vi "DT Read Encode.vi"(11 "Reset Encoders":bool) -> (2 "Drivetrain Encoder Values":T1)   [LabVIEW 2017]
uses:
  Common Code/Drivetrain Encoder Values.ctl
  Common Code/DT Encoder Values.ctl
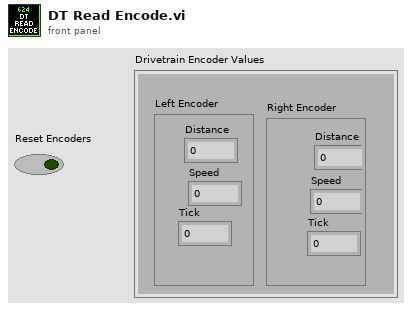
[diagram p1: front panel]
types:
  T1 = typedef "Drivetrain Encoder Values.ctl" = cluster{"Left Encoder":cluster{"Distance":dbl, "Speed":dbl, "Tick":dbl}, "Right Encoder":cluster{"Distance":dbl, "Speed":dbl, "Tick":dbl}}
  T2 = typedef "DT Encoder Values.ctl" = cluster{"Left Encoder":cluster{"Distance":dbl, "Speed":dbl, "Tick":dbl}, "Right Encoder":cluster{"Distance":dbl, "Speed":dbl, "Tick":dbl}}
  T3 = typedef "WPI_EncoderDevRef.ctl" = cluster{"DevStatus":errorcluster, "EncoderIndex":T4, "CounterIndex":T5, "DistancePerCount":dbl, "Decoding Type":T6}
  T4 = typedef "FPGA_EncoderIdx.ctl" = enum8{"Enc 0", "Enc 1", "Enc 2", "Enc 3", "Enc 4", "Enc 5", "Enc 6", "Enc 7", "Invalid"}
  T5 = typedef "FPGA_CounterCtrSystemIndex.ctl" = enum8{"Ctr 0", "Ctr 1", "Ctr 2", "Ctr 3", "Ctr 4", "Ctr 5", "Ctr 6", "Ctr 7", "Invalid"}
  T6 = typedef "WPI_EncoderType.ctl" = enum16{"1x", "2x", "4x"}
  T7 = typedef "Encoder Values.ctl" = cluster{"Distance":dbl, "Speed":dbl, "Tick":dbl}
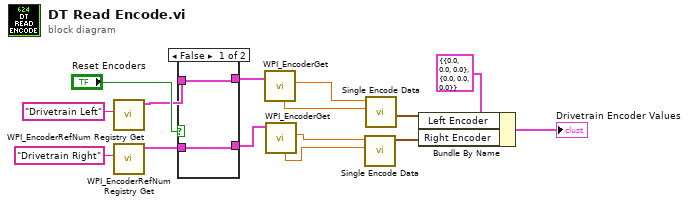
[diagram p0: block diagram]
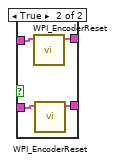
[diagram p2: hidden frame]
diagram:
  n1 = call <vilib>:"WPI_EncoderRefNum Registry Get.vi"("refnum name"="Drivetrain Left") -> ("EncoderDevRef"=w12:T3)  [unwired: 9 in, 1 out]
  n2 = call <vilib>:"WPI_EncoderRefNum Registry Get.vi"("refnum name"="Drivetrain Right") -> ("EncoderDevRef"=w11:T3)  [unwired: 9 in, 1 out]
  n3 = case shown="False" "Reset Encoders" {
    tunnel: w12 -> [w17 w21]
    tunnel: w11 -> [w16 w20]
    tunnel: [w17 w19] -> w10
    tunnel: [w16 w18] -> w9
    frame False {
    }
    frame True {
      n4 = call <vilib>:"WPI_EncoderReset.vi"("EncoderDevRef"=w21) -> ("EncoderDevRef"=w19:T3)  [unwired: 9 in, 1 out]
      n5 = call <vilib>:"WPI_EncoderReset.vi"("EncoderDevRef"=w20) -> ("EncoderDevRef"=w18:T3)  [unwired: 9 in, 1 out]
    }
  }
  n6 = call <vilib>:"WPI_EncoderGet.vi"("EncoderDevRef"=w10) -> ("Distance"=w5:dbl, "Rate"=w6:dbl)  [unwired: 5 in, 4 out]
  n7 = call <vilib>:"WPI_EncoderGet.vi"("EncoderDevRef"=w9) -> ("Distance"=w7:dbl, "Rate"=w8:dbl)  [unwired: 5 in, 4 out]
  n8 = call "Single Encode Data.vi"("Rate"=w8, "Distance"=w7) -> ("Encoder Values"=w2:T7)  [unwired: 9 in]
  n9 = call "Single Encode Data.vi"("Rate"=w6, "Distance"=w5) -> ("Encoder Values"=w3:T7)  [unwired: 9 in]
  n10 = Bundle By Name(cluster=T2 {"Left Encoder"={"Distance"=0.0, "Speed"=0.0, "Tick"=0.0}, "Right Encoder"={"Distance"=0.0, "Speed"=0.0, "Tick"=0.0}} ("Drivetrain Encoder Values"), "Left Encoder"=w3, "Right Encoder"=w2) -> (→"Drivetrain Encoder Values":T2)
